vi "Read Value.vi"(8 "error in (no error)":errorcluster, 11 "Quick-GUI-Update in":refnum<class "Quick-GUI-Update.lvclass">) -> (0 "error out":errorcluster, 3 "Quick-GUI-Update out":refnum<class "Quick-GUI-Update.lvclass">)   [LabVIEW 2020, in "Quick-GUI-Update.lvclass"]
uses:
  Quick-GUI-Update.lvclass
  Quick-GUI-Update.lvclass/Quick-GUI-Update.ctl
panel:
  out "Status":u8[](array[numeric])
  in  "Value In":variant
  in  "Lable":string
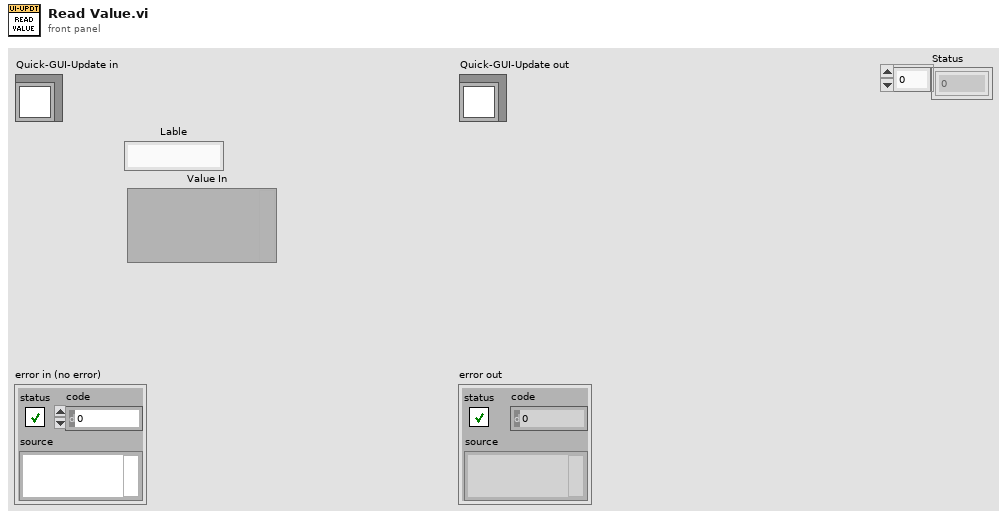
[diagram p1: front panel]
types:
  T1 = map{string, set{cluster{"Ctrl-Ref":refnum<vi>, "Ctrl Index":i32, "Class-Name":string}}}
  T2 = set{cluster{"Ctrl-Ref":refnum<vi>, "Ctrl Index":i32, "Class-Name":string}}
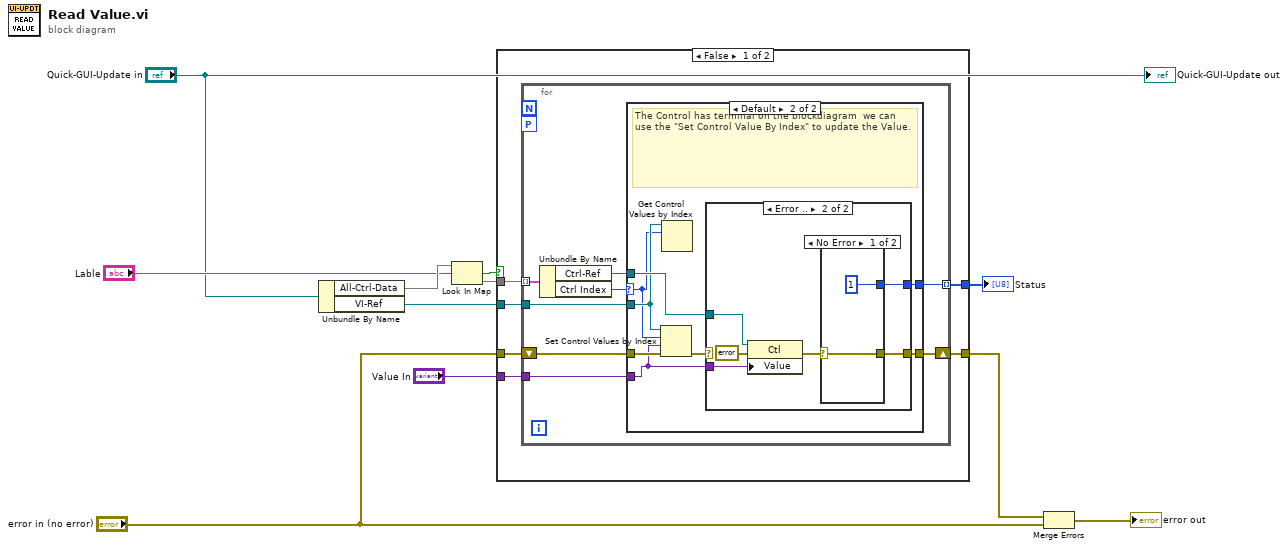
[diagram p0: block diagram]
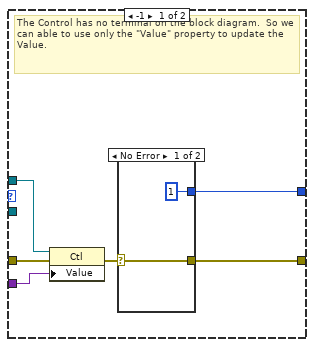
[diagram p2: hidden frame]
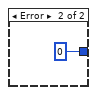
[diagram p3: hidden frame]
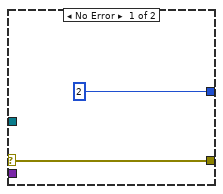
[diagram p4: hidden frame]
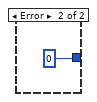
[diagram p5: hidden frame]
diagram:
  n1 = Unbundle By Name("Quick-GUI-Update in") -> ("All-Ctrl-Data"=w10:T1, "VI-Ref"=w6:refnum<vi>)
  n2 = Look In Map(map=w10, key="Lable") -> (key not found?=w8:bool, value=w7:T2)  [unwired: 1 in]
  n3 = case shown="False" w8 {
    tunnel: "error in (no error)" -> [w15 w54]
    tunnel: "Value In" -> [w16 _]
    tunnel: w7 -> [w12 _]
    tunnel: w6 -> [w17 _]
    tunnel: [w14 w54] -> w4
    tunnel: [w13 _] -> w5
    frame False {
      n4 = for {
        tunnel: w12 -> [w23] mode=indexing
        tunnel: w17 -> [w19]
        tunnel: w16 -> [w22]
        shift-right: [w20] -> w14
        shift-left: w15 -> [w21]
        tunnel: [w18] -> w13 mode=indexing
        workers-P: _ -> [_]
        n5 = Unbundle By Name(w23) -> ("Ctrl-Ref"=w24:refnum<vi>, "Ctrl Index"=w25:i32)
        n6 = case shown="Default" w25 {
          selector: w25 -> [_ w35]
          tunnel: w24 -> [w31 w41]
          tunnel: w22 -> [w30 w38]
          tunnel: w21 -> [w29 w40]
          tunnel: [w26 w39] -> w20
          tunnel: w19 -> [_ w36]
          tunnel: [w28 w37] -> w18
          frame -1 {
            # "The Control has no terminal on the block diagram.  So we can able to use only the \"Value\" property to update the Value."
            n7 = property class="Ctl"(reference=w31, error in=w29, "Value"=w30) -> (error out=w27:errorcluster)  [unwired: 1 out]
            n8 = case shown="No Error" w27 {
              selector: w27 -> [w32 _]
              tunnel: [u8 1 u8 0] -> w28
              tunnel: [w32 _] -> w26
              frame No Error {
              }
              frame Error {
              }
            }
          }
          frame Default {
            # "The Control has terminal on the blockdiagram  we can use the \"Set Control Value By Index\" to update the Value."
            n9 = Set Control Values by Index(0:w36, 1:w35, 2:w38, 3:w40) -> (11:w42:errorcluster)
            n10 = Get Control Values by Index(0:w36, 1:w35) -> ()  [unwired: 1 in, 2 out]
            n11 = case shown="Error .." w42 {
              selector: w42 -> [w44 _]
              tunnel: [w44 w45] -> w39
              tunnel: w41 -> [_ w50]
              tunnel: w38 -> [_ w49]
              tunnel: [u8 2 w47] -> w37
              frame No Error {
              }
              frame Error {
                n12 = property class="Ctl"(reference=w50, error in=errorcluster {"status"=FALSE, "code"=0, "source"=""} ("error in (no error)"), "Value"=w49) -> (error out=w46:errorcluster)  [unwired: 1 out]
                n13 = case shown="No Error" w46 {
                  selector: w46 -> [w51 _]
                  tunnel: [u8 1 u8 0] -> w47
                  tunnel: [w51 _] -> w45
                  frame No Error {
                  }
                  frame Error {
                  }
                }
              }
            }
          }
        }
      }
    }
    frame True {
    }
  }
  "Status" <- w5
  n14 = Merge Errors(w4, "error in (no error)") -> (→"error out":errorcluster)
  "Quick-GUI-Update out" <- "Quick-GUI-Update in"
